vi "Set Resolution.vi"(8 "error in (no error)":errorcluster, 10 "Front Panel Window:Window Bounds":T1={"Left"=0, "Top"=0, "Right"=1920, "Bottom"=1080}, 11 "VI in":refnum<vi>) -> (0 "error out":errorcluster, 3 "VI out":refnum<vi>)   [LabVIEW 2018]
uses:
  <vilib>/Utility/miscctls.llb/LVRectTypeDef.ctl
panel:
  # "1920"
  # "1080"
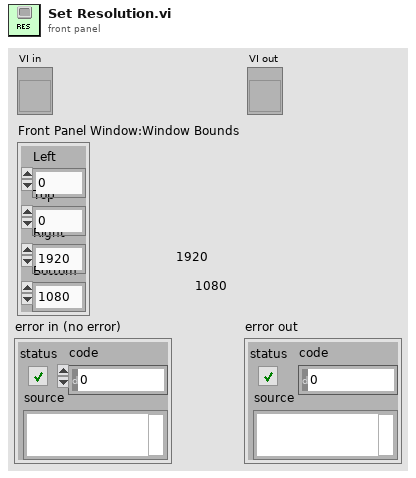
[diagram p1: front panel]
types:
  T1 = typedef "LVRectTypeDef.ctl" = cluster{"Left":i16, "Top":i16, "Right":i16, "Bottom":i16}
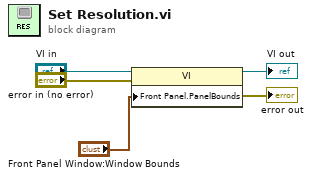
[diagram p0: block diagram]
diagram:
  n1 = property class="VI"(reference="VI in", error in="error in (no error)", "Front Panel.PanelBounds"="Front Panel Window:Window Bounds") -> (reference out=→"VI out":refnum<vi>, error out=→"error out":errorcluster)
